vi "Latch.vi"(1 "reset":bool, 2 "set":bool) -> (0 "latch":bool)   [LabVIEW 2014]
panel:
  # "Boolian latch"
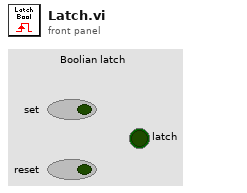
[diagram p1: front panel]
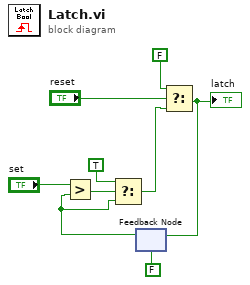
[diagram p0: block diagram]
diagram:
  n1 = feedback #1(FALSE ("latch")) -> (w2:bool)
  n2 = Greater?(x="set", y=w2) -> (0:w6:bool)
  n3 = Select(t=TRUE ("latch"), s=w6, f=w2) -> (s? t:f=w4:bool)
  n4 = Select(t=FALSE ("latch"), s="reset", f=w4) -> (s? t:f=w3:bool)
  "latch" <- w3
  n5 = feedback-in #1(w3) -> ()
